vi "Get Server Internal UEs.vi"(11 "OOP Server in":refnum<class "HVC9.lvclass">) -> (2 "Server Internal UEs":T1, 3 "OOP Server out":refnum<class "HVC9.lvclass">)   [LabVIEW 2019, in "HVC9.lvlib" / "HVC9.lvclass"]
uses:
  HVC9.lvclass
  typeDefs/Server Internal UEs.ctl
  typeDefs/Server Internal Message.ctl
  HVC9.lvclass/HVC9.ctl
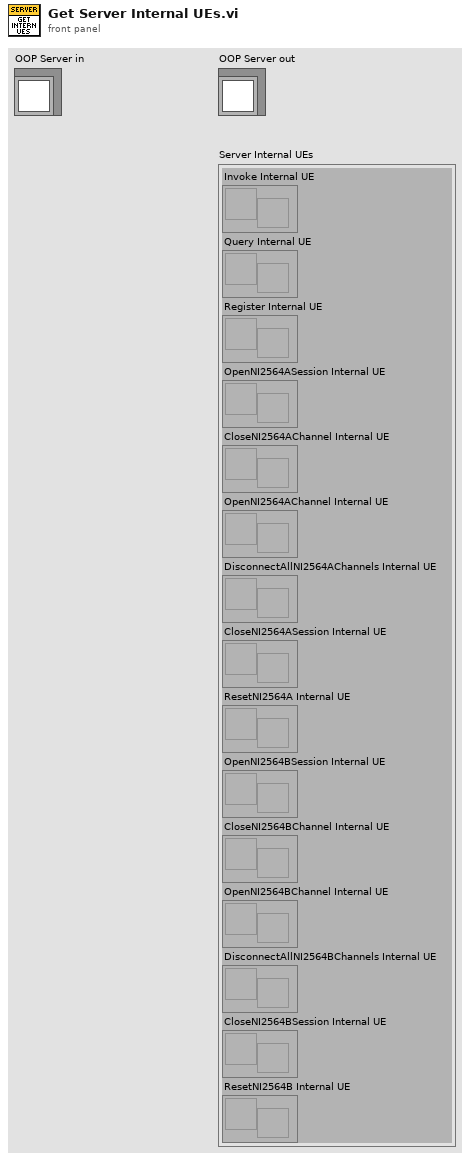
[diagram p1: front panel]
types:
  T1 = typedef "HVC9.lvlib/HVC9.lvclass/Server Internal UEs.ctl" = cluster{"Invoke Internal UE":refnum<user-event>, "Query Internal UE":refnum<user-event>, "Register Internal UE":refnum<user-event>, "OpenNI2564ASession Internal UE":refnum<user-event>, "CloseNI2564AChannel Internal UE":refnum<user-event>, "OpenNI2564AChannel Internal UE":refnum<user-event>, "DisconnectAllNI2564AChannels Internal UE":refnum<user-event>, "CloseNI2564ASession Internal UE":refnum<user-event>, "ResetNI2564A Internal UE":refnum<user-event>, "OpenNI2564BSession Internal UE":refnum<user-event>, "CloseNI2564BChannel Internal UE":refnum<user-event>, "OpenNI2564BChannel Internal UE":refnum<user-event>, "DisconnectAllNI2564BChannels Internal UE":refnum<user-event>, "CloseNI2564BSession Internal UE":refnum<user-event>, "ResetNI2564B Internal UE":refnum<user-event>}
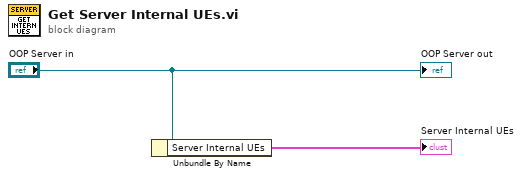
[diagram p0: block diagram]
diagram:
  n1 = Unbundle By Name("OOP Server in") -> ("Server Internal UEs"=→"Server Internal UEs":T1)
  "OOP Server out" <- "OOP Server in"
